vi "Filter & Build DependentTypeDefs&Parents.vi"(11 "Dependendent TypeDefs wParents":T1[](array[typedef])) -> (3 "Filtered Dependendent TypeDefs wParents":T1[](array[typedef]))   [LabVIEW 2013, in "DiscoverCommonTypeDefCallers.lvlib"]
doc: "This VI takes an array of clusters, and appends a new cluster to the array, if and only if the new TypeDef name does NOT already exist as a cluster element in the array; thus preventing duplicates. Furthermore, if the TypeDef name DOES already exist, a new parent name will be appended to the nested array of parent names, if and only if the new parent name does NOT already exist in that particular nested array; thus preventing duplicate parent names within each cluster. The end result is an array of unique TypeDef names, each bundled with an array of unique parent (caller) names."
uses:
  DiscoverCommonTypeDefCallers.lvlib
  Controls/DependendentTypeDefwParents.ctl
panel:
  in  "Dependendent TypeDef wParents":T1
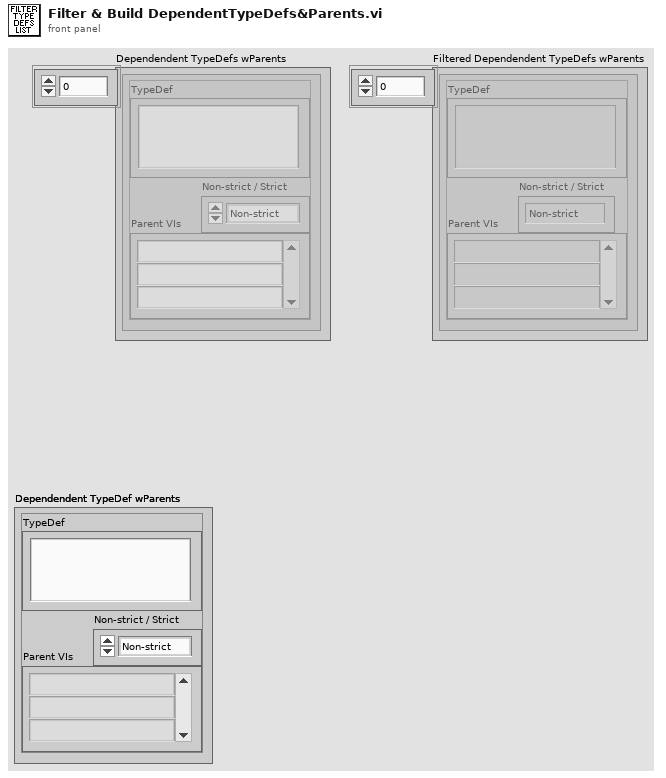
[diagram p1: front panel]
types:
  T1 = typedef "DiscoverCommonTypeDefCallers.lvlib/DependendentTypeDefwParents.ctl" = cluster{"TypeDef":string, "Non-strict / Strict":enum32{"Non-strict", "Strict"}, "Parent VIs":string[]}
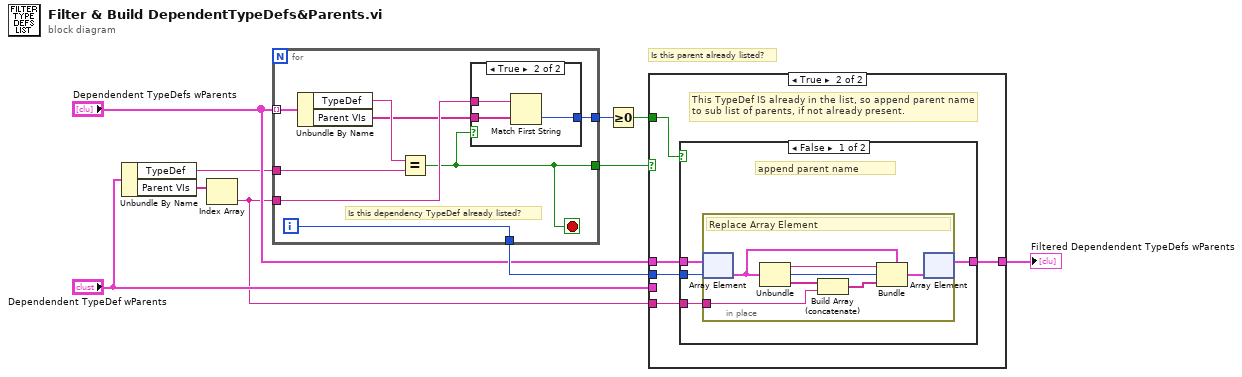
[diagram p0: block diagram]
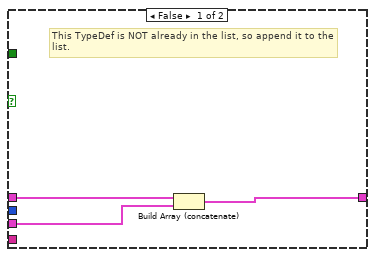
[diagram p2: hidden frame]
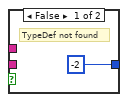
[diagram p4: hidden frame]
diagram:
  # "Is this parent already listed?"
  n1 = Unbundle By Name("Dependendent TypeDef wParents") -> ("TypeDef"=w3:string, "Parent VIs"=w2:string[])
  n2 = Index Array(array=w2) -> (element=w1:string)  [unwired: 1 in]
  n3 = for {
    tunnel: "Dependendent TypeDefs wParents" -> [w15] mode=indexing
    tunnel: w1 -> [w18]
    tunnel: w3 -> [w17]
    tunnel: [w11] -> w9
    tunnel: [w14] -> w8
    tunnel: [w12] -> w6
    i -> [w12]
    stop <- w11 stop-if-true
    # "Is this dependency TypeDef already listed?"
    n4 = Unbundle By Name(w15) -> ("TypeDef"=w16:string, "Parent VIs"=w13:string[])
    n5 = Equal?(x=w16, y=w17) -> (x = y?=w11:bool)
    n6 = case shown="True" w11 {
      tunnel: w13 -> [_ w22]
      tunnel: w18 -> [_ w21]
      tunnel: [-2 ("index") w20] -> w14
      frame False {
        # "TypeDef not found"
      }
      frame True {
        n7 = Match First String(2:w22, 3:w21) -> (0:w20:i32)  [unwired: 1 out]
      }
    }
  }
  n8 = Greater Or Equal To 0?(x=w8) -> (x >= 0?=w7:bool)
  n9 = case shown="True" w9 {
    tunnel: "Dependendent TypeDefs wParents" -> [w24 w29]
    tunnel: [w25 w28] -> w10
    tunnel: "Dependendent TypeDef wParents" -> [w23 _]
    tunnel: w6 -> [_ w26]
    tunnel: w1 -> [_ w27]
    tunnel: w7 -> [_ w30]
    frame False {
      # "This TypeDef is NOT already in the list, so append it to the list."
      n10 = Build Array (concatenate)(w24, w23) -> (w25:T1[])
    }
    frame True {
      # "This TypeDef IS already in the list, so append parent name to sub list of parents, if not already present."
      n11 = case shown="False" w30 {
        tunnel: w29 -> [w34 w42]
        tunnel: [w33 w42] -> w28
        tunnel: w27 -> [w31 _]
        tunnel: w26 -> [w32 _]
        frame False {
          # "append parent name"
          n12 = in-place {
            in-place-border: w31 -> [w41]
            # "Replace Array Element"
            n13 = in-place-array #1(w34, w32) -> (w38:T1)
            n14 = Unbundle(w38) -> ("TypeDef"=w40:string, "Non-strict / Strict"=w35:enum32{"Non-strict", "Strict"}, "Parent VIs"=w36:string[])
            n15 = Build Array (concatenate)(w36, w41) -> (w37:string[])
            n16 = Bundle(cluster=w38, "TypeDef"=w40, "Non-strict / Strict"=w35, "Parent VIs"=w37) -> (w39:T1)
            n17 = in-place-array #1(w39) -> (w33:T1[])  [unwired: 1 out]
          }
        }
        frame True {
          # "parent name is already present"
        }
      }
    }
  }
  "Filtered Dependendent TypeDefs wParents" <- w10
